vi "Conductus Set PID.vi"(2 "PID param":dbl[][](array[numeric])=[[1.0, 0.0, 0.0, 0.0], [1.0, 0.0, 0.0, 0.0]] format="%.3f", 3 "Instrument Address":refnum<visa-resource-name>) -> (0 "Stop":bool)   [LabVIEW 2020]
doc: "Reads the PID paramters of the Conductus temperature controller. The output is an array consisting P, I, D, and P0. The input is the numeric GPIB address.\nScott Hannahs, NHMFL, November 1996"
panel:
  # "P"
  # "I"
  # "D"
  # "P0"
  # "Heater"
  # "Analog"
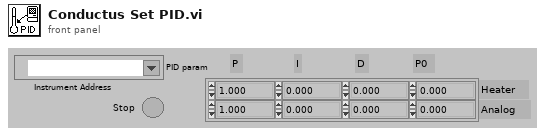
[diagram p1: front panel]
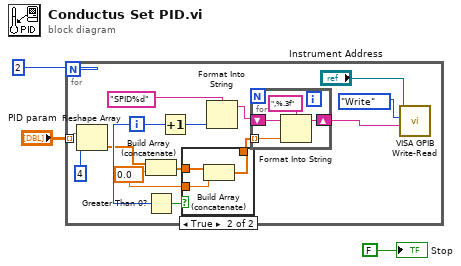
[diagram p0: block diagram]
diagram:
  n1 = for {
    N: 2 -> [_]
    tunnel: "PID param" -> [w14] mode=indexing
    i -> [w16]
    w11 = 0.0 ("Input Element")
    n2 = Reshape Array(w14, 4 ("Dimension Size")) -> (w7:dbl[])
    n3 = Build Array (concatenate)(w7, w11) -> (w8:dbl[])
    n4 = Greater Than 0?(x=w16) -> (x > 0?=w10:bool)
    n5 = Increment(x=w16) -> (x+1=w17:i32)
    n6 = case shown="True" w10 {
      tunnel: [w18 w20] -> w9
      tunnel: w8 -> [w18 w21]
      tunnel: w11 -> [_ w19]
      frame False {
      }
      frame True {
        n7 = Build Array (concatenate)(w21, w19) -> (w20:dbl[])
      }
    }
    n8 = Format Into String(format string="SPID%d", w17) -> (resulting string=w12:string)  [unwired: 2 in, 1 out]
    n9 = for {
      tunnel: w9 -> [w25] mode=indexing
      shift-right: [w22] -> w4
      shift-left: w12 -> [w23]
      n10 = Format Into String(format string=",%.3f", initial string=w23, w25) -> (resulting string=w22:string)  [unwired: 1 in, 1 out]
    }
    n11 = call "VISA GPIB Write-Read.vi"("Command"=w4, "Action"=enum16{"Write", "Read", "Write & Read"}."Write", "VISA resource name"="Instrument Address") -> ()  [unwired: 5 in, 4 out]
  }
  "Stop" <- FALSE ("Stop")
